vi "VP.vi"(0 "VPStates":refnum<vi>, 1 "Processes":refnum<vi>, 2 "INP":refnum<vi>, 3 "PORTS":refnum<vi>, 4 "OUTPUT VARS":refnum<vi>, 5 "VPOutputMsgs":refnum<vi>, 6 "OUTP":refnum<vi>, 7 "INPUT VARS":refnum<vi>, 8 "VP2GUI":refnum<vi>, 9 "States":refnum<vi>) -> ()   [LabVIEW 2019]
uses:
  lib/Ports.lvclass
panel:
  out "Здачения 3":string[](array[string])
  out "Типы 3":string[](array[string])
  out "Output:":string[](array[string])
  out "Value:":string[](array[string])
  out "Type::":string[](array[string])
  out "Input:":string[](array[string])
  out "Output messages":T1(array[cluster])
  out "States of processes:":string[][](table)
  in  "OUT Ports Array 3":cluster{"Port":string, "Value":bool[]}[](array[cluster])
  in  "INP Ports Array":cluster{"Port\nPort":string, "Value":bool[]}[](array[cluster])
  # "Virtual plant"
  # "Global variables"
  # "Алгоритм управления"
  # "Input ports values"
  # "Значения входных портов"
  # "Output ports values"
  # "Значения выходных портов"
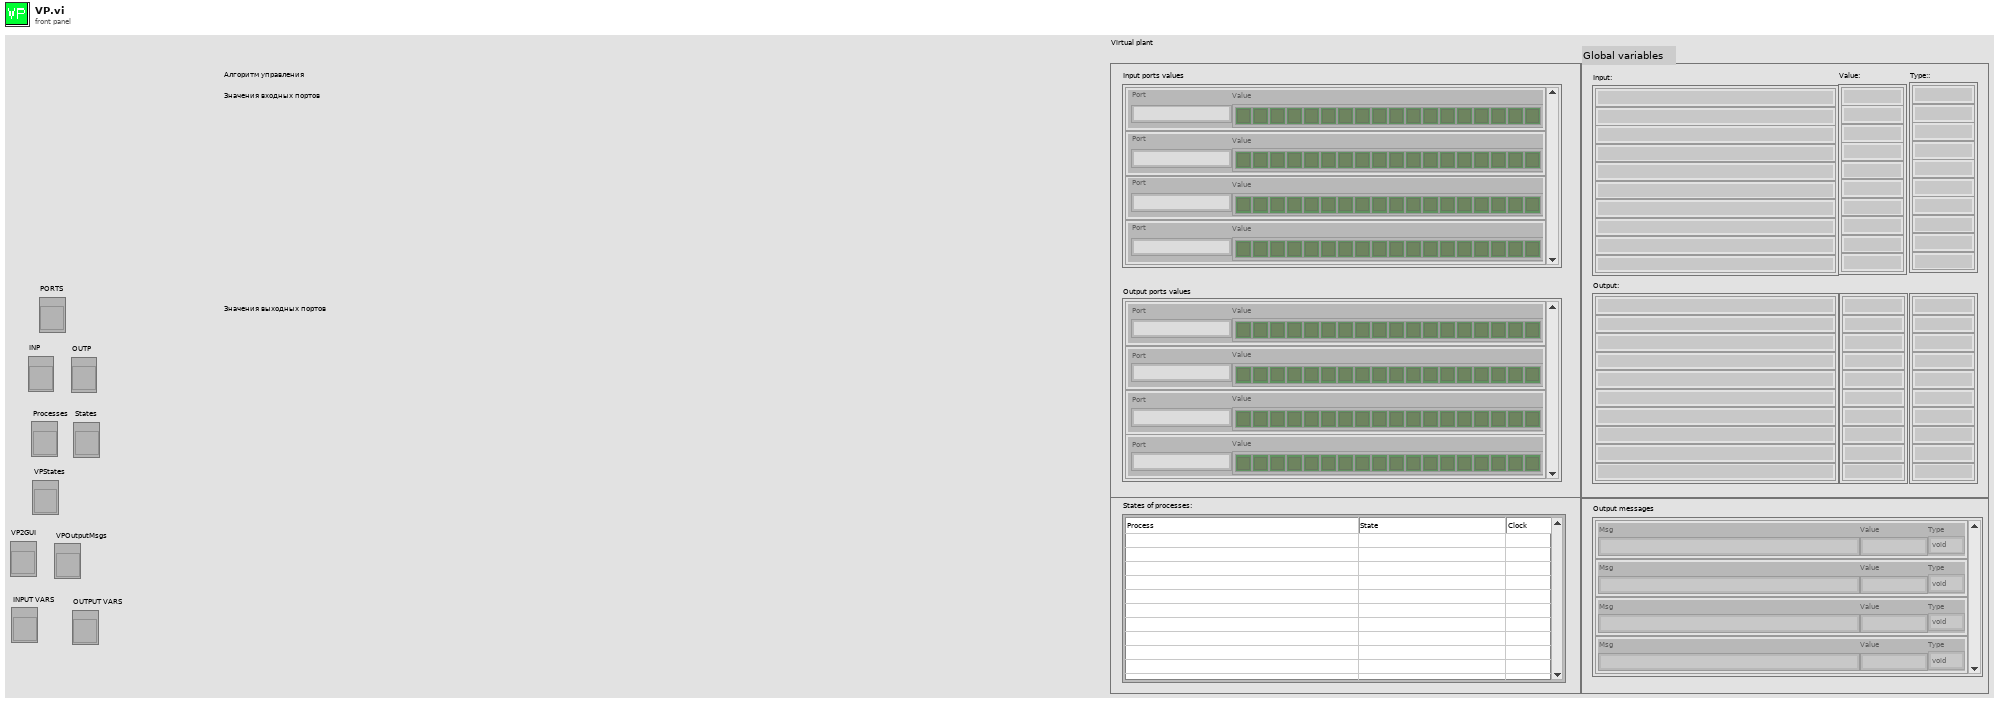
[diagram p1: front panel]
types:
  T1 = cluster{"Msg":string, "Value":string, "Type":enum16{"void", "byte", "int", "float"}}[]
  T2 = cluster{"Сообщение":string, "Значение":string, "Тип":enum16{"void", "byte", "int", "float"}}
  T3 = cluster{"Input varables names":string[], "Input varables type":string[], "Input varables ports":i32[], "Input varables bytes":i32[]}
  T4 = cluster{"Output varables names":string[], "Output varables type":string[], "Output varables ports":i32[], "Output varables bytes":i32[]}
  T5 = cluster{"CA Output Numbers ":i32[], "CA Input Numbers":i32[], "VP Input Names":string[], "VP Output Names ":string[]}
  T6 = cluster{"Сообщение":string, "Значение":string, "Тип":enum16{"void", "byte", "int", "float"}}[]
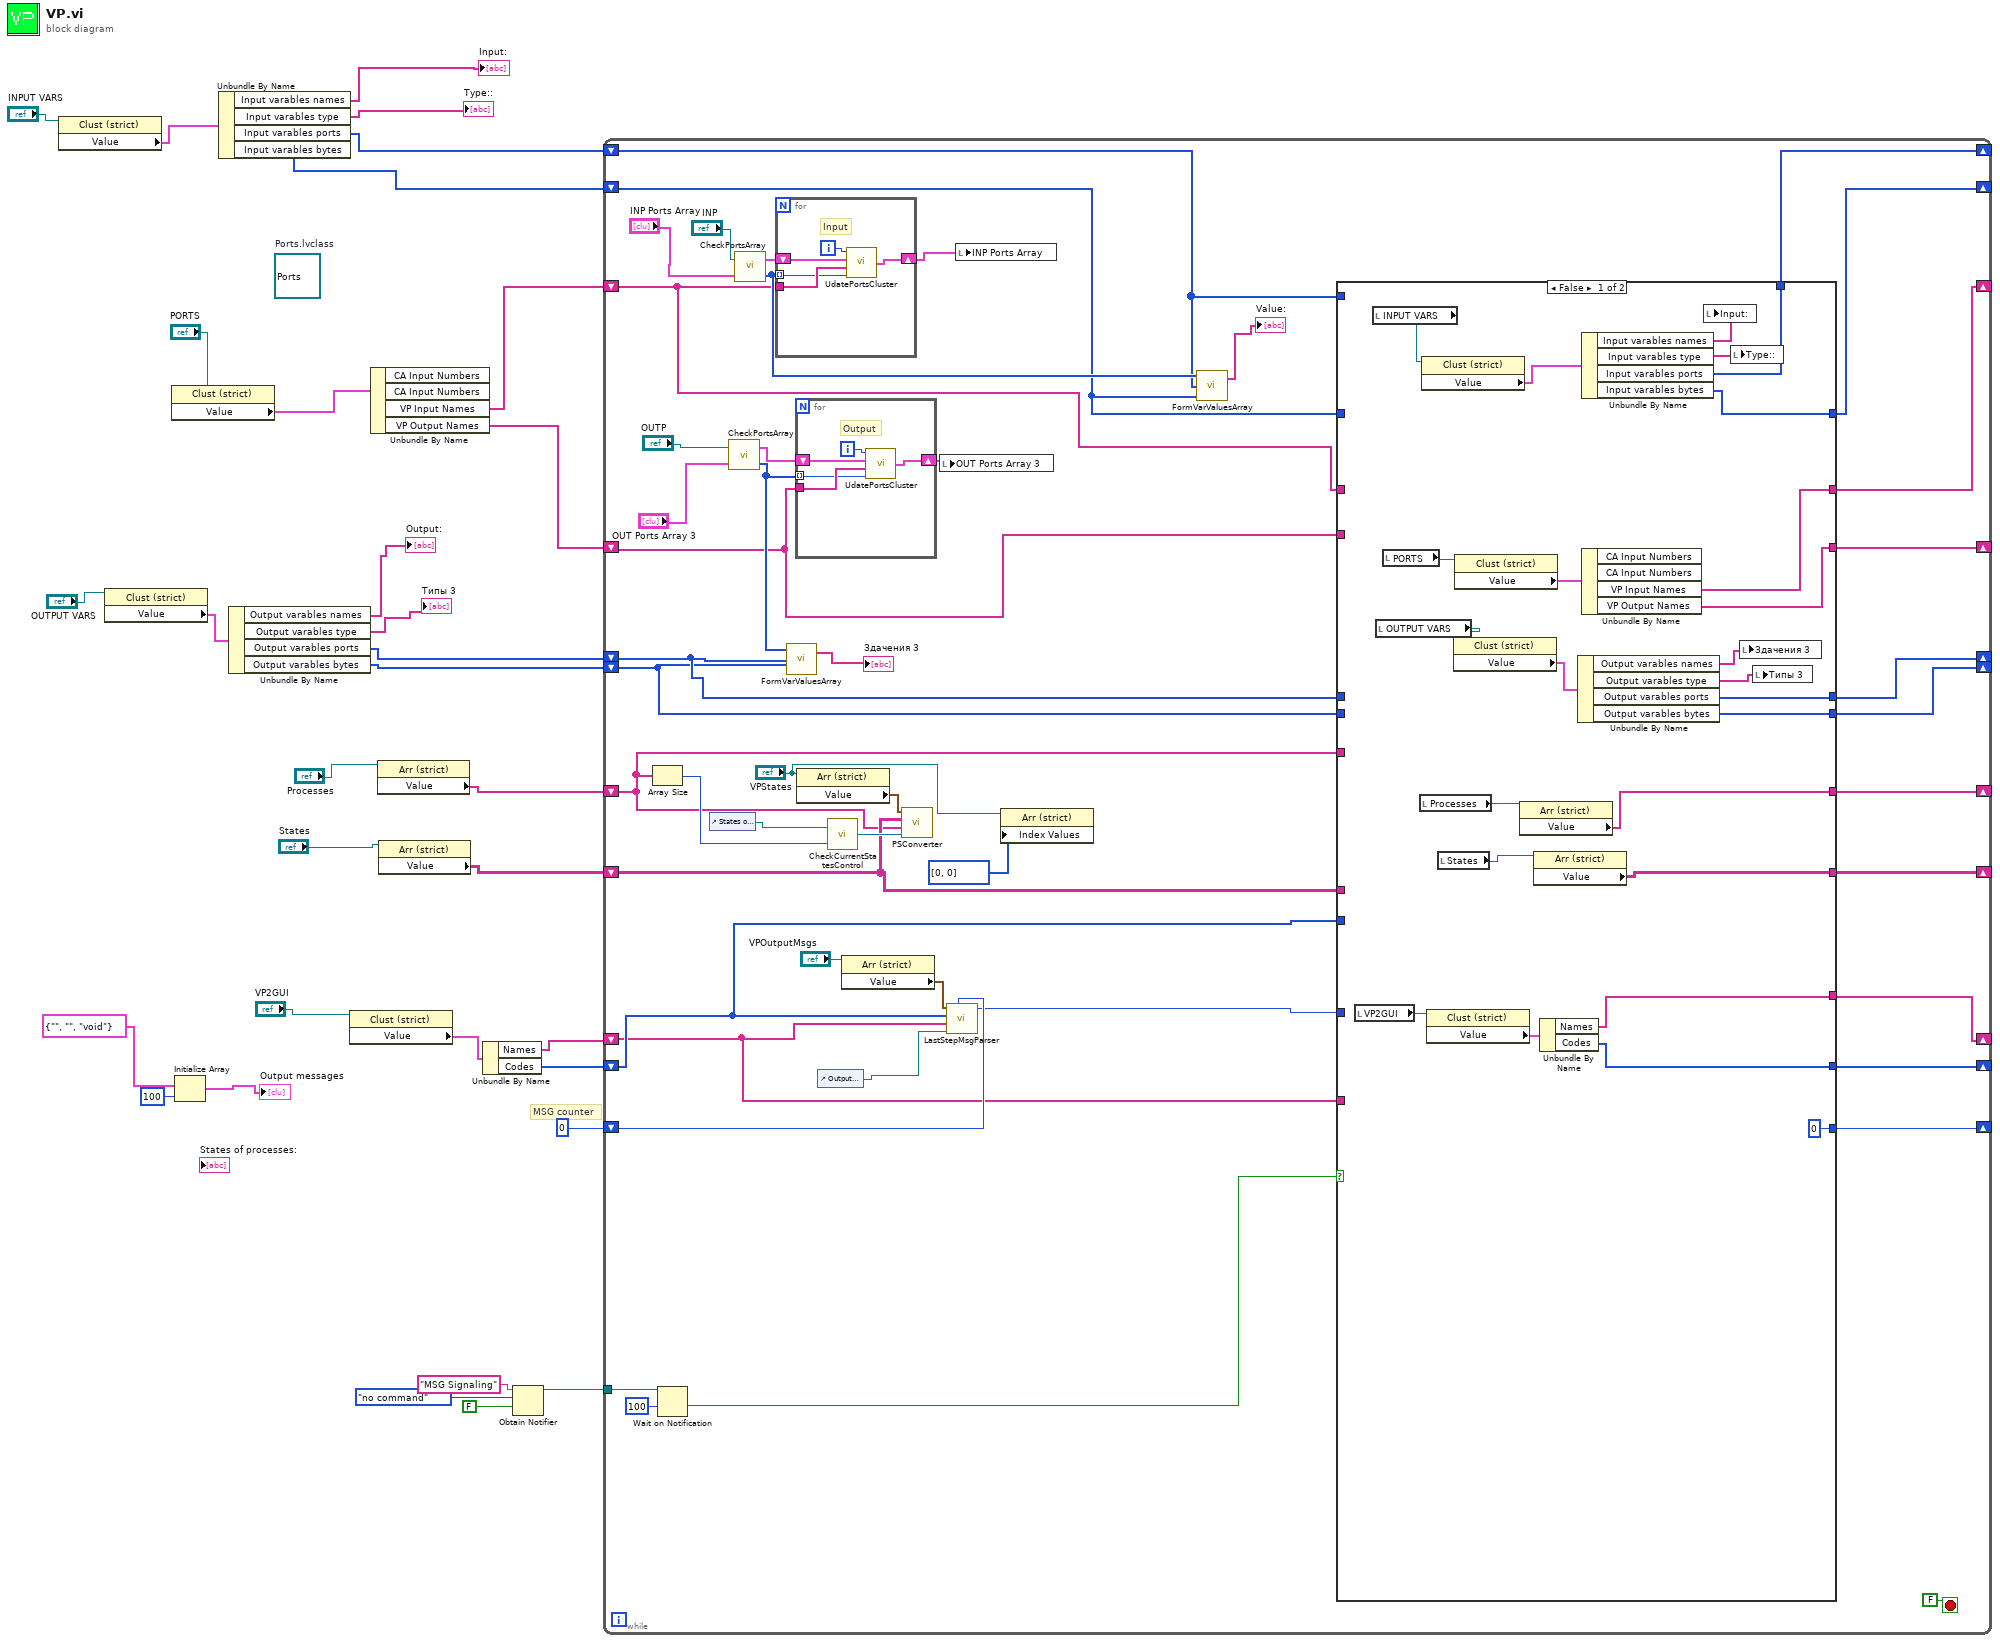
[diagram p0: block diagram]
diagram:
  (unwired) refnum<class "Ports.lvclass"> refnum  # Ports.lvclass
  # "MSG counter"
  n1 = property class="Clust (strict)"(reference="INPUT VARS") -> ("Value"=w17:T3)  [unwired: 1 in, 2 out]
  n2 = property class="Clust (strict)"(reference="OUTPUT VARS") -> ("Value"=w12:T4)  [unwired: 1 in, 2 out]
  n3 = property class="Clust (strict)"(reference="PORTS") -> ("Value"=w31:T5)  [unwired: 1 in, 2 out]
  n4 = Initialize Array(T2 {"Сообщение"="", "Значение"="", "Тип"=enum."void"} ("Cluster"), 100 ("dimension size")) -> (→"Output messages":T6)
  n5 = Unbundle By Name(w17) -> ("Input varables names"=→"Input:":string[], "Input varables type"=→"Type::":string[], "Input varables ports"=w16:i32[], "Input varables bytes"=w15:i32[])
  n6 = Unbundle By Name(w12) -> ("Output varables names"=→"Output:":string[], "Output varables type"=→"Типы 3":string[], "Output varables ports"=w11:i32[], "Output varables bytes"=w10:i32[])
  n7 = property class="Clust (strict)"(reference="VP2GUI") -> ("Value"=w24:cluster{"Names":string[], "Codes":i32[]})  [unwired: 1 in, 2 out]
  n8 = Unbundle By Name(w31) -> ("VP Input Names"=w30:string[], "VP Output Names"=w14:string[])  [unwired: 2 out]
  n9 = property class="Arr (strict)"(reference="Processes") -> ("Value"=w27:string[])  [unwired: 1 in, 2 out]
  n10 = property class="Arr (strict)"(reference="States") -> ("Value"=w26:string[][])  [unwired: 1 in, 2 out]
  n11 = Unbundle By Name(w24) -> ("Names"=w23:string[], "Codes"=w22:i32[])
  n12 = Obtain Notifier(name (unnamed)="MSG Signaling", notification data type=enum16{"no command", "refresh"}."no command", create if not found? (T)=FALSE) -> (notifier out=w6:refnum<notifier>)  [unwired: 1 in, 2 out]
  n13 = while {
    shift-right: [w62] -> _
    shift-left: 0 ("dimension size") -> [w68]
    tunnel: w6 -> [w65]
    shift-right: [w60] -> _
    shift-left: w22 -> [w61]
    shift-right: [w59] -> _
    shift-left: w23 -> [w58]
    shift-right: [w53] -> _
    shift-left: w26 -> [w56]
    shift-right: [w54] -> _
    shift-left: w27 -> [w55]
    shift-right: [w45] -> _
    shift-left: w15 -> [w51]
    shift-right: [w46] -> _
    shift-left: w16 -> [w52]
    shift-right: [w48] -> _
    shift-left: w14 -> [w49]
    shift-right: [w47] -> _
    shift-left: w30 -> [w50]
    shift-right: [w38] -> _
    shift-left: w11 -> [w36]
    shift-right: [w37] -> _
    shift-left: w10 -> [w35]
    stop <- FALSE ("stop") stop-if-true
    n14 = Array Size(array=w55) -> (size(s)=w57:i32)
    n15 = Wait on Notification(notifier=w65, timeout in ms (-1)=100) -> (timed out?=w64:bool)  [unwired: 2 in, 3 out]
    n16 = control-ref of="States of processes:"() -> (w42:refnum<vi>)
    n17 = call "CheckPortsArray.vi"("INP Ports Array 2"="OUT Ports Array 3", "INP"="OUTP") -> ("Value"=w66:i8[], "INP Ports Array"=w77:cluster{"String":string, "Array 2":bool[]}[])
    n18 = call "CheckPortsArray.vi"("INP Ports Array 2"="INP Ports Array", "INP"="INP") -> ("Value"=w67:i8[], "INP Ports Array"=w79:cluster{"String":string, "Array 2":bool[]}[])
    n19 = for {
      tunnel: w67 -> [w125] mode=indexing
      tunnel: w50 -> [w126]
      shift-right: [w122] -> w43
      shift-left: w79 -> [w123]
      i -> [w124]
      # "Input"
      n20 = call "UdatePortsCluster.vi"("Numeric 2"=w125, "Input Names"=w126, "Ports Array"=w123, "index"=w124) -> ("INP Ports Array 2"=w122:cluster{"String":string, "Array 2":bool[]}[])
    }
    n21 = call "FormVarValuesArray.vi"("varables bytes"=w35, "varables ports"=w36, "Ports"=w66) -> ("Values Array"=→"Здачения 3":string[])  [unwired: 1 in]
    n22 = for {
      tunnel: w66 -> [w120] mode=indexing
      tunnel: w49 -> [w121]
      shift-right: [w117] -> w76
      shift-left: w77 -> [w118]
      i -> [w119]
      # "Output"
      n23 = call "UdatePortsCluster.vi"("Numeric 2"=w120, "Input Names"=w121, "Ports Array"=w118, "index"=w119) -> ("INP Ports Array 2"=w117:cluster{"String":string, "Array 2":bool[]}[])
    }
    n24 = property class="Arr (strict)"(reference="VPStates") -> ("Value"=w75:cluster{"TimeInState":u16, "cur_state":i8}[])  [unwired: 1 in, 2 out]
    n25 = control-ref of="Output messages"() -> (w41:refnum<vi>)
    n26 = call "CheckCurrentStatesControl.vi"("Processes"=w57, "Inp reference"=w42) -> ("Out Refnum"=w74:refnum<vi>)
    n27 = property class="Arr (strict)"(reference="VPOutputMsgs") -> ("Value"=w69:cluster{"MSG":i16, "param":i32, "Type":i16}[])  [unwired: 1 in, 2 out]
    n28 = call "PSConverter.vi"("Tbl Refnum"=w74, "PROC"=w55, "STATES"=w56, "Input claster"=w75) -> ()  [unwired: 1 out]
    n29 = local write "OUT Ports Array 3"(w76) -> ()
    n30 = call "LastStepMsgParser.vi"("Arr Refnum"=w41, "Out MSG Names"=w58, "old msg counter"=w68, "Codes"=w61, "Msg Array"=w69) -> ("current msg counter"=w63:i32)  [unwired: 4 in, 1 out]
    n31 = local write "INP Ports Array"(w43) -> ()
    n32 = property class="Arr (strict)"(reference="VPStates", "Index Values"=u32[] [0, 0]) -> ()  [unwired: 1 in, 2 out]
    n33 = call "FormVarValuesArray.vi"("varables bytes"=w51, "varables ports"=w52, "Ports"=w67) -> ("Values Array"=→"Value:":string[])  [unwired: 1 in]
    n34 = case shown="False" w64 {
      tunnel: w63 -> [_ w114]
      tunnel: [0 ("current msg counter") w114] -> w62
      tunnel: w61 -> [_ w116]
      tunnel: [w101 w116] -> w60
      tunnel: [w102 w115] -> w59
      tunnel: w58 -> [_ w115]
      tunnel: w56 -> [_ w106]
      tunnel: w55 -> [_ w107]
      tunnel: [w99 w107] -> w54
      tunnel: [w97 w106] -> w53
      tunnel: w49 -> [_ w113]
      tunnel: w52 -> [_ w111]
      tunnel: w51 -> [_ w110]
      tunnel: w50 -> [_ w112]
      tunnel: [w94 w113] -> w48
      tunnel: [w93 w112] -> w47
      tunnel: [w90 w111] -> w46
      tunnel: [w89 w110] -> w45
      tunnel: [w82 w109] -> w38
      tunnel: [w81 w108] -> w37
      tunnel: w36 -> [_ w109]
      tunnel: w35 -> [_ w108]
      frame False {
        n35 = local read "VP2GUI"() -> (w104:refnum<vi>)
        n36 = local read "INPUT VARS"() -> (w91:refnum<vi>)
        n37 = local read "OUTPUT VARS"() -> (w85:refnum<vi>)
        n38 = local read "PORTS"() -> (w95:refnum<vi>)
        n39 = local read "Processes"() -> (w100:refnum<vi>)
        n40 = property class="Clust (strict)"(reference=w91) -> ("Value"=w92:T3)  [unwired: 1 in, 2 out]
        n41 = property class="Clust (strict)"(reference=w104) -> ("Value"=w103:cluster{"Names":string[], "Codes":i32[]})  [unwired: 1 in, 2 out]
        n42 = local read "States"() -> (w98:refnum<vi>)
        n43 = property class="Clust (strict)"(reference=w85) -> ("Value"=w86:T4)  [unwired: 1 in, 2 out]
        n44 = property class="Clust (strict)"(reference=w95) -> ("Value"=w96:T5)  [unwired: 1 in, 2 out]
        n45 = property class="Arr (strict)"(reference=w100) -> ("Value"=w99:string[])  [unwired: 1 in, 2 out]
        n46 = property class="Arr (strict)"(reference=w98) -> ("Value"=w97:string[][])  [unwired: 1 in, 2 out]
        n47 = Unbundle By Name(w103) -> ("Names"=w102:string[], "Codes"=w101:i32[])
        n48 = Unbundle By Name(w86) -> ("Output varables names"=w84:string[], "Output varables type"=w83:string[], "Output varables ports"=w82:i32[], "Output varables bytes"=w81:i32[])
        n49 = Unbundle By Name(w92) -> ("Input varables names"=w88:string[], "Input varables type"=w87:string[], "Input varables ports"=w90:i32[], "Input varables bytes"=w89:i32[])
        n50 = Unbundle By Name(w96) -> ("VP Input Names"=w93:string[], "VP Output Names"=w94:string[])  [unwired: 2 out]
        n51 = local write "Input:"(w88) -> ()
        n52 = local write "Type::"(w87) -> ()
        n53 = local write "Здачения 3"(w84) -> ()
        n54 = local write "Типы 3"(w83) -> ()
      }
      frame True {
      }
    }
  }
